vi "Get Most Recent Frame (if active).vi"(8 "error in (no error)":errorcluster, 11 "Photometrics Camera in":refnum<class "Photometrics Camera.lvclass">) -> (0 "error out":errorcluster, 3 "Photometrics Camera out":refnum<class "Photometrics Camera.lvclass">)   [LabVIEW 2023, in "Photometrics Camera.lvlib" / "Photometrics Camera.lvclass"]
uses:
  Photometrics Camera.lvclass
  C:/FlashGordon/Development/Hardware/Camera/Camera.lvclass
  C:/Program Files/National Instruments/LabVIEW 2023/vi.lib/ActorFramework/Actor/Actor.lvclass
  Users/Public/Documents/Photometrics/TPM-LabVIEWSamples BETA/TPM LabVIEW adapter/SDK/Controls/Acquisition Status.ctl
  Users/Public/Documents/Photometrics/TPM-LabVIEWSamples BETA/TPM LabVIEW adapter/SDK/Controls/Region Index.ctl
  <vilib>/ActorFramework/Actor/Actor.lvclass/Actor.ctl
  Application Messages/New Frame Notify Msg/New Frame Notify Msg.lvclass/New Frame Notify Msg.ctl
  <vilib>/ActorFramework/Message Enqueuer/Message Enqueuer.lvclass/Message Enqueuer.ctl
  <vilib>/ActorFramework/Message Enqueuer/Enqueue.vi
  Application Messages/New Frame Notify Msg/New Frame Notify Msg.lvclass
  C:/Program Files/National Instruments/LabVIEW 2023/vi.lib/ActorFramework/Message/Message.lvclass
  Resources/GLOBAL/GLOBAL Time-critical.vi
  <vilib>/ActorFramework/Message Priority Queue/Priority Enqueue.vi
  Photometrics Camera.lvclass/Photometrics Camera.ctl
  <vilib>/ActorFramework/Actor/Actor.lvclass
  Camera/Camera.lvlib
  Users/Public/Documents/Photometrics/TPM-LabVIEWSamples BETA/TPM LabVIEW adapter/Camera/Camera.lvclass
panel:
  out "Disk Streaming Failed":bool[](array[boolean])
  out "size(s)":i32[](array[numeric])
  out "output array":u16[][][](array[numeric])
  out "CapturedFrames":i32
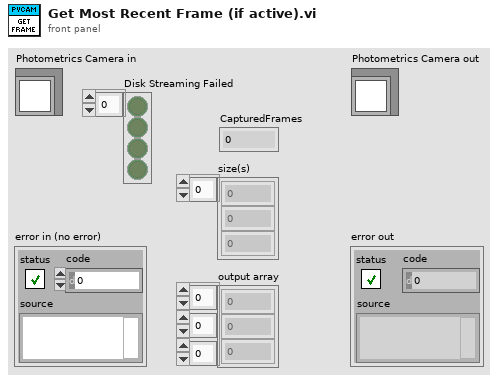
[diagram p1: front panel]
types:
  T1 = typedef "Acquisition Status.ctl" = enum32{"Idle", "Starting", "Acquiring", "Stopping"}
  T2 = typedef "Physical Camera Assignment.ctl" = cluster{"Channel Name":string, "Serial Number":string, "Flip Vertically":bool, "Flip Horizontally":bool, "photonsPerCount":dbl, "wavelength":i16}
  T3 = typedef "Frames Captured.ctl" = u64
  T4 = typedef "Region Index.ctl" = i32
  T5 = typedef "Camera Regions.ctl" = T6[]
  T6 = typedef "Region.ctl" = cluster{"Origin X":u16, "Origin Y":u16, "Width":u16, "Height":u16}
  T7 = cluster{"Origin X":dbl, "Origin Y":dbl, "Width":dbl, "Height":dbl}
  T8 = cluster{"Origin X":u16, "Origin Y":u16, "Width":u16, "Height":u16}
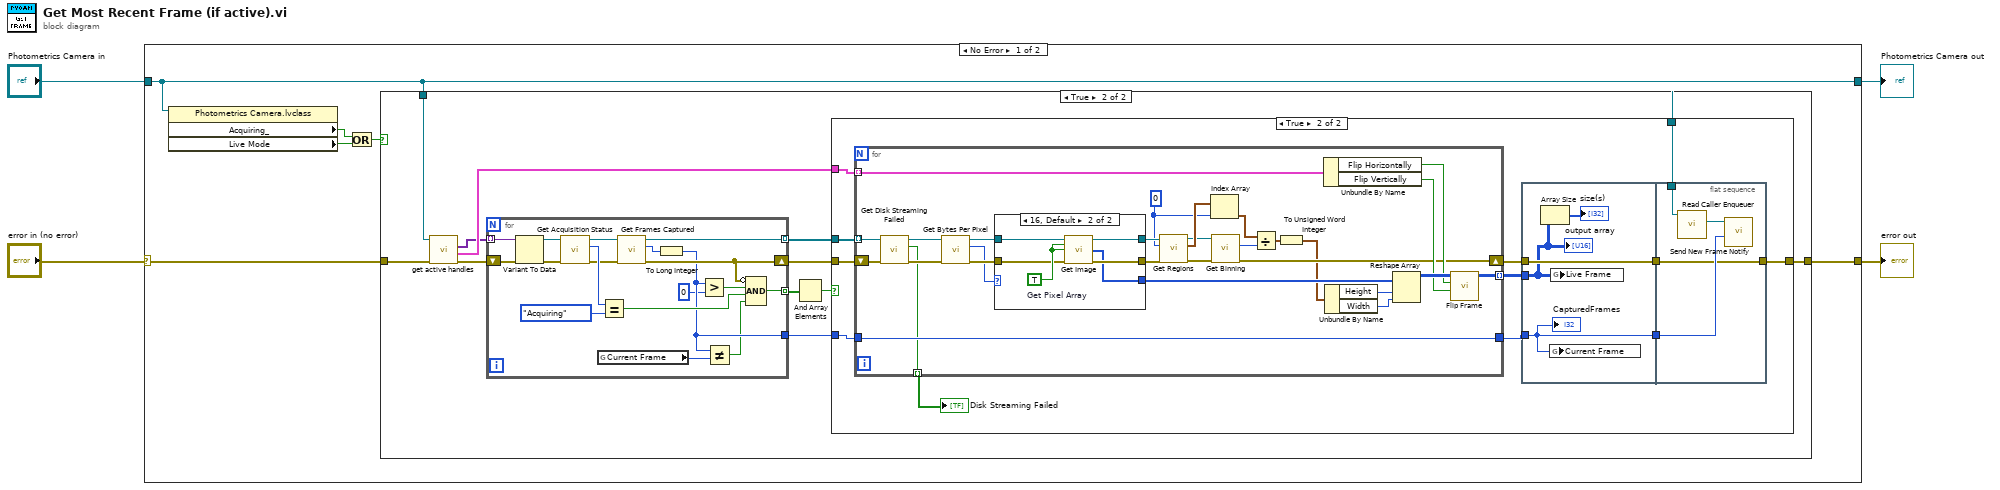
[diagram p0: block diagram]
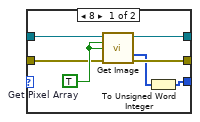
[diagram p4: hidden frame]
diagram:
  n1 = case shown="No Error" "error in (no error)" {
    selector: "error in (no error)" -> [w10 w104]
    tunnel: [w9 w104] -> w2
    tunnel: "Photometrics Camera in" -> [w8 w103]
    tunnel: [w8 w103] -> w1
    frame No Error {
      n2 = property class="Photometrics Camera.lvclass"(reference=w8) -> ("Acquiring_"=w5:bool, "Live Mode"=w7:bool)  [unwired: 1 in, 2 out]
      n3 = Or(x=w5, y=w7) -> (x .or. y?=w6:bool)
      n4 = case shown="True" w6 {
        tunnel: w10 -> [w11 w19]
        tunnel: [w11 w18] -> w9
        tunnel: w8 -> [_ w17]
        frame False {
        }
        frame True {
          n5 = call-dynamic "get active handles.vi"("error in (no error)"=w19, "Camera in"=w17) -> ("error out"=w15:errorcluster, "Active Cameras"=w16:T2[], "Handles"=w12:variant[])  [unwired: 5 in, 2 out]
          n6 = for {
            tunnel: [w32] -> w22 mode=indexing
            shift-right: [w29] -> w20
            shift-left: w15 -> [w37]
            tunnel: [w33] -> w14 mode=indexing
            tunnel: [w26] -> w13
            tunnel: w12 -> [w28] mode=indexing
            n7 = Variant To Data(error in=w37, Variant=w28) -> (data=w38:refnum<class "Camera.lvclass">, error out=w36:errorcluster)  [unwired: 1 in]
            n8 = call "Get Acquisition Status.vi"("error in (no error)"=w36, "Camera in"=w38) -> ("error out"=w34:errorcluster, "Acquisition Status"=w40:T1, "Camera out"=w35:refnum<class "Camera.lvclass">)  [unwired: 7 in]
            n9 = global read "GLOBAL Time-critical.vi" "Current Frame"() -> (w24:i32)
            n10 = Equal?(x=w40, y=Acquisition_Status."Acquiring" ("Acquisition Status")) -> (x = y?=w31:bool)
            n11 = call "Get Frames Captured.vi"("error in (no error)"=w34, "Camera in"=w35) -> ("error out"=w29:errorcluster, "Frames Captured"=w27:T3, "Camera out"=w33:refnum<class "Camera.lvclass">)  [unwired: 7 in]
            n12 = To Long Integer(number=w27) -> (32bit integer=w26:i32)
            n13 = Greater?(x=w26, y=0) -> (0:w30:bool)
            n14 = Not Equal?(x=w26, y=w24) -> (x != y?=w23:bool)
            n15 = Compound Arithmetic op=AND(invert w29, w30, w31, w23) -> (w32:bool)
          }
          n16 = And Array Elements(Boolean array=w22) -> (logical AND=w21:bool)
          n17 = case shown="True" w21 {
            tunnel: w20 -> [w41 w53]
            tunnel: [w41 w50] -> w18
            tunnel: w17 -> [_ w46]
            tunnel: w16 -> [_ w45]
            tunnel: w14 -> [_ w44]
            tunnel: w13 -> [_ w43]
            frame False {
            }
            frame True {
              n18 = for {
                shift-right: [w73] -> w51
                shift-left: w53 -> [w63]
                tunnel: [w84] -> w49 mode=indexing
                tunnel: [w68] -> w48
                tunnel: w45 -> [w87] mode=indexing
                tunnel: w44 -> [w64] mode=indexing
                tunnel: w43 -> [w68]
                tunnel: [w62] -> w42 mode=indexing
                w67 = T4 0 ("Region Index")
                n19 = call "Get Disk Streaming Failed.vi"("error in (no error)"=w63, "Camera in"=w64) -> ("error out"=w65:errorcluster, "Disk Streaming Failed"=w62:bool, "Camera out"=w66:refnum<class "Camera.lvclass">)  [unwired: 7 in]
                n20 = call "Get Bytes Per Pixel.vi"("error in (no error)"=w65, "Camera in"=w66) -> ("error out"=w83:errorcluster, "Bytes Per Pixel"=w81:u32, "Camera out"=w82:refnum<class "Camera.lvclass">)  [unwired: 7 in]
                n21 = case shown="16, Default" w81 {
                  tunnel: w83 -> [w94 w100]
                  tunnel: [w92 w98] -> w89
                  tunnel: [w93 w99] -> w79
                  tunnel: w82 -> [w95 w101]
                  tunnel: [w90 w97] -> w80
                  frame 8 {
                    w96 = TRUE  # Get Pixel Array
                    n22 = call "Get Image.vi"("Camera in"=w95, "Get Image (T)"=w96, "Get Pixel Array (F)"=w96, "error in (no error)"=w94) -> ("Camera out"=w90:refnum<class "Camera.lvclass">, "Pixels UNS8"=w91:u8[], "error out"=w93:errorcluster)  [unwired: 6 in, 3 out]
                    n23 = To Unsigned Word Integer(number=w91) -> (unsigned 16bit integer=w92:u16[])
                  }
                  frame 16, Default {
                    w102 = TRUE  # Get Pixel Array
                    n24 = call "Get Image.vi"("Camera in"=w101, "Get Image (T)"=w102, "Get Pixel Array (F)"=w102, "error in (no error)"=w100) -> ("Camera out"=w97:refnum<class "Camera.lvclass">, "Pixels UNS16"=w98:u16[], "error out"=w99:errorcluster)  [unwired: 6 in, 3 out]
                  }
                }
                n25 = call "Get Regions.vi"("error in (no error)"=w79, "Region Index"=w67, "Camera in"=w80) -> ("error out"=w74:errorcluster, "Camera Regions"=w78:T5, "Camera out"=w75:refnum<class "Camera.lvclass">)  [unwired: 6 in]
                n26 = Index Array(array=w78, index=w67) -> (element=w71:T6)
                n27 = call "Get Binning.vi"("error in (no error)"=w74, "Camera in"=w75) -> ("error out"=w73:errorcluster, "Binning X"=w72:u16)  [unwired: 6 in, 2 out]
                n28 = Divide(x=w71, y=w72) -> (x/y=w70:T7)
                n29 = To Unsigned Word Integer(number=w70) -> (unsigned 16bit integer=w69:T8)
                n30 = Unbundle By Name(w87) -> ("Flip Horizontally"=w86:bool, "Flip Vertically"=w85:bool)
                n31 = Unbundle By Name(w69) -> ("Height"=w77:u16, "Width"=w76:u16)
                n32 = Reshape Array(w89, w77, w76) -> (w88:u16[][])
                n33 = call "Flip Frame.vi"("Flip Vertically"=w85, "Flip Horizontally"=w86, "Input Array"=w88) -> ("output array"=w84:u16[][])  [unwired: 8 in]
              }
              "Disk Streaming Failed" <- w42
              n34 = flat-sequence {
                tunnel: w51 -> [w57]
                tunnel: [w57] -> w52
                tunnel: w49 -> [w55]
                tunnel: w48 -> [w56]
                tunnel: [w56] -> w47
                tunnel: w52 -> [w59]
                tunnel: [w59] -> w50
                tunnel: w47 -> [w60]
                tunnel: w46 -> [w61]
                frame #0 {
                  n35 = Array Size(array=w55) -> (size(s)=→"size(s)":i32[])
                  n36 = global write "GLOBAL Time-critical.vi" "Current Frame"(w56) -> ()
                  n37 = global write "GLOBAL Time-critical.vi" "Live Frame"(w55) -> ()
                  "CapturedFrames" <- w56
                  "output array" <- w55
                }
                frame #1 {
                  n38 = call <vilib>:"Read Caller Enqueuer.vi"("Actor"=w61) -> ("Caller Enqueuer"=w58:refnum<class "Message Enqueuer.lvclass">)  [unwired: 10 in]
                  n39 = call "Send New Frame Notify.vi"("Frame Number\n(starts with 1)"=w60, "Message Enqueuer"=w58) -> ()  [unwired: 8 in, 2 out]
                }
              }
            }
          }
        }
      }
    }
    frame Error {
    }
  }
  "error out" <- w2
  "Photometrics Camera out" <- w1
